vi "Demo Process.vi"() -> ()   [LabVIEW 2020]
panel:
  out "DblStatus 4":cluster{"Color":u32, "Value":dbl}
  out "DblStatus 3":cluster{"Color":u32, "Value":dbl}
  out "DblStatus 2":cluster{"Color":u32, "Value":dbl}
  out "DblStatus":cluster{"Color":u32, "Value":dbl}
  in  "2WayH 4":cluster{"Picture":picture, "Command":bool}={"Picture"=bytes[9690], "Command"=FALSE}
  in  "2WayV":cluster{"Picture":picture, "Command":bool}={"Picture"=bytes[9690], "Command"=FALSE}
  in  "2WayH 3":cluster{"Picture":picture, "Command":bool}={"Picture"=bytes[9690], "Command"=FALSE}
  in  "2WayH 2":cluster{"Picture":picture, "Command":bool}={"Picture"=bytes[9690], "Command"=FALSE}
  in  "2WayH":cluster{"Picture":picture, "Command":bool}={"Picture"=bytes[9690], "Command"=FALSE}
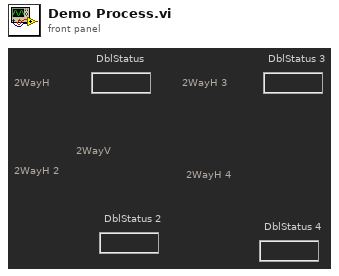
[diagram p1: front panel]
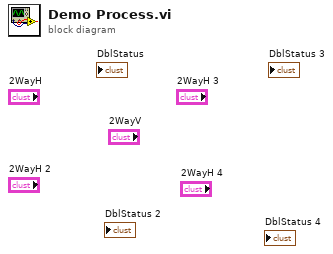
[diagram p0: block diagram]
diagram:
